vi "VISA XYStage.vi"() -> ()   [LabVIEW 2013]
panel:
  in  "XY-STAGE bytes":u32=70
  in  "XY-STAGE maskT":u16=128
  in  "XY-STAGE item tag":string[](array[string])
  in  "XY-STAGE expected reply":string[](array[string])
  in  "XY-STAGE command":string[](array[string])
  in  "XY-STAGE reply terminator":string="\n"
  in  "XY-STAGE termination char\n(0xA = '\\n' = LF)":u8=13
  in  "XY-STAGE command terminator":string="\r"
  in  "XY-STAGE mask":u16=64
  in  "XY-STAGE VISA resource name":refnum<visa-resource-name>="COM10"
  in  "XY-STAGE stop bits":u16(ring)=20 items=["1.0"=10, "1.5"=15, "2.0"=20]
  in  "XY-STAGE flow control":u16(ring) items=["None", "XON/XOFF", "RTS/CTS", "XON/XOFF & RTS/CTS", "DTR/DSR", "XON/XOFF & DTR/DSR"]
  in  "XY-STAGE parity":enum16{"None", "Odd", "Even", "Mark", "Space"}(ring)
  in  "XY-STAGE data bits":u16=8
  in  "XY-STAGE baud rate":u32=9600
  # "XY-STAGE VISA"
  # "VISA Configuration"
  # "ASI com4\nLudl com9"
  # "ASI 1.0 stop  bits\nLudl 2.0 stolp bits"
  # "VISA Flush Buffer"
  # "ASI \\r\nLudl \\r"
  # "ASI \\r\\n\nLudl \\n"
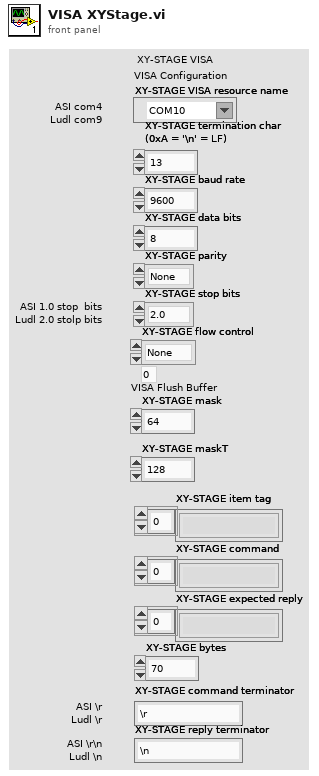
[diagram p1: front panel]
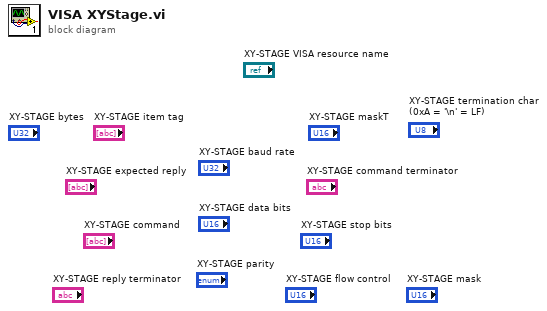
[diagram p0: block diagram]
diagram:
